vi "S2C_PCIe7841_Proc_GetClusterValues.vi"(4 "LabelText":string, 6 "Cmd In":string, 8 "Error In":errorcluster, 9 "CtrlRef":refnum<vi>) -> (0 "Error Out":errorcluster, 1 "Cmd Out":string, 2 "Send?":bool, 3 "Settings":string[][](array[string]))   [LabVIEW 2015]
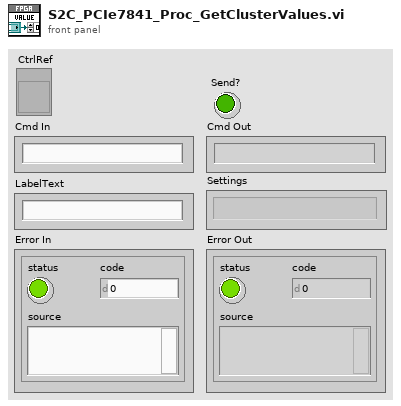
[diagram p1: front panel]
types:
  T1 = cluster{"Bit0":bool, "Bit1":bool, "Bit2":bool, "Bit3":bool, "Bit4":bool, "Bit5":bool, "Bit6":bool, "Bit7":bool, "Send":bool, "Size":bool, "State":bool}
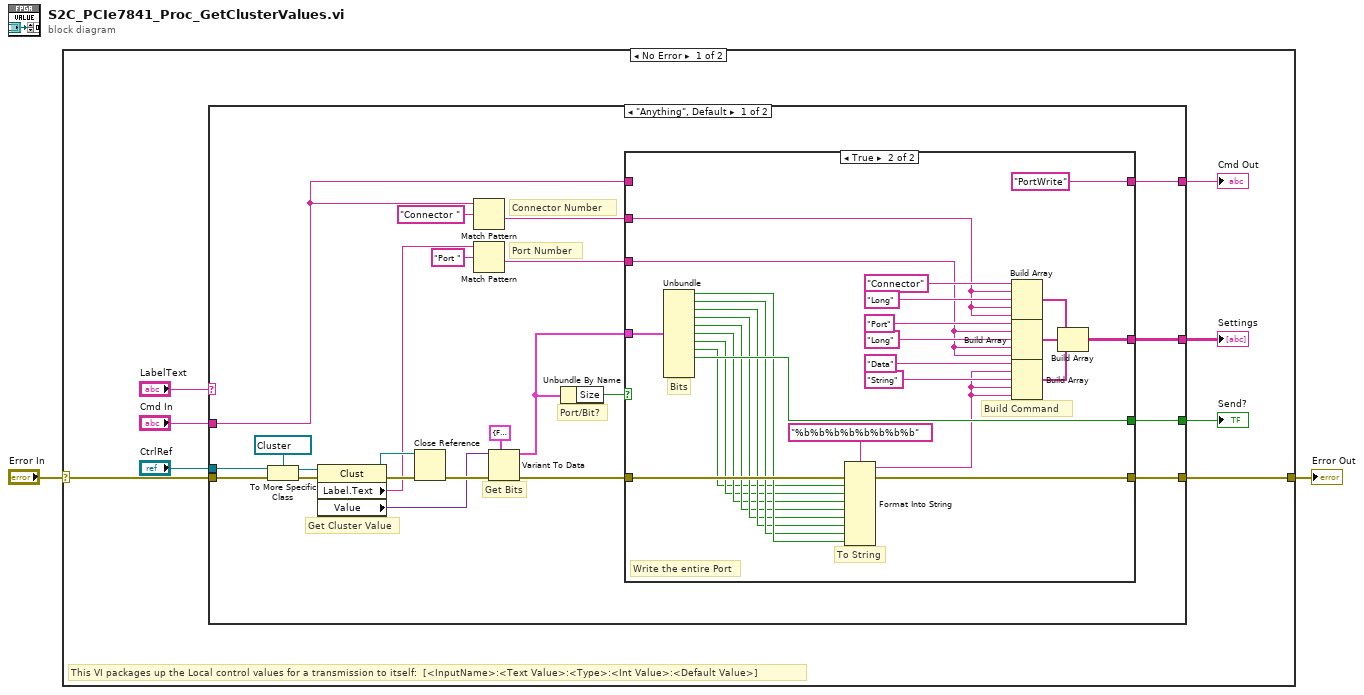
[diagram p0: block diagram]
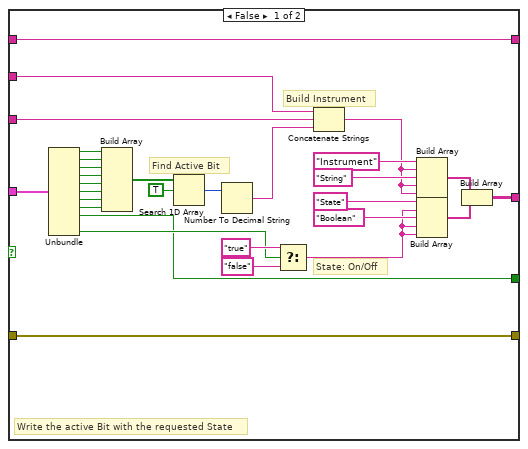
[diagram p2: hidden frame]
diagram:
  n1 = case shown="No Error" "Error In" {
    selector: "Error In" -> [w9 w92]
    tunnel: [w10 w92] -> w1
    frame No Error {
      # "This VI packages up the Local control values for a transmission to itself:  [<InputName>:<Text Value>:<Type>:<Int Value>:<Default Value>]"
      n2 = case shown="\"Anything\", Default" "LabelText" {
        tunnel: [w13 w91] -> w10
        tunnel: w9 -> [w33 w91]
        tunnel: "CtrlRef" -> [w32 _]
        tunnel: [w18 _] -> w7
        tunnel: [w17 _] -> w6
        tunnel: "Cmd In" -> [w12 _]
        tunnel: [w11 _] -> w3
        frame "Anything", Default {
          # "Port/Bit?"
          # "Get Bits"
          # "Connector Number"
          # "Port Number"
          # "Get Cluster Value"
          n3 = To More Specific Class(target class=refnum<vi> refnum ("reference"), reference=w32, error in=w33) -> (specific class reference=w30:refnum<vi>, error out=w31:errorcluster)
          n4 = property class="Clust"(reference=w30, error in=w31) -> (reference out=w28:refnum<vi>, error out=w29:errorcluster, "Label.Text"=w24:string, "Value"=w25:variant)
          n5 = Close Reference(reference=w28, error in (no error)=w29) -> (error out=w26:errorcluster)
          n6 = Match Pattern(string=w12, regular expression="Connector ") -> (after substring=w20:string)  [unwired: 1 in, 3 out]
          n7 = Match Pattern(string=w24, regular expression="Port ") -> (after substring=w19:string)  [unwired: 1 in, 3 out]
          n8 = Variant To Data(error in=w26, type=T1 {"Bit0"=FALSE, "Bit1"=FALSE, "Bit2"=FALSE, "Bit3"=FALSE, "Bit4"=FALSE, "Bit5"=FALSE, "Bit6"=FALSE, "Bit7"=FALSE, "Send"=FALSE, "Size"=FALSE, "State"=FALSE} ("Port 1"), Variant=w25) -> (data=w16:T1, error out=w14:errorcluster)
          n9 = Unbundle By Name(w16) -> ("Size"=w15:bool)
          n10 = case shown="True" w15 {
            tunnel: w16 -> [w62 w89]
            tunnel: w20 -> [w34 w82]
            tunnel: w19 -> [w35 w81]
            tunnel: [w40 w84] -> w18
            tunnel: [w38 w83] -> w17
            tunnel: w14 -> [w37 w78]
            tunnel: [w37 w76] -> w13
            tunnel: w12 -> [w36 _]
            tunnel: [w36 "PortWrite" ("Cmd In")] -> w11
            frame False {
              # "Write the active Bit with the requested State"
              # "State: On/Off"
              # "Find Active Bit"
              # "Build Instrument"
              n11 = Unbundle(w62) -> ("Bit0"=w54:bool, "Bit1"=w55:bool, "Bit2"=w56:bool, "Bit3"=w57:bool, "Bit4"=w58:bool, "Bit5"=w59:bool, "Bit6"=w60:bool, "Bit7"=w61:bool, "Send"=w38:bool, "State"=w39:bool)  [unwired: 1 out]
              n12 = Build Array(w54, w55, w56, w57, w58, w59, w60, w61) -> (w53:bool[])
              n13 = Search 1D Array(1D array=w53, element=TRUE) -> (index of element=w51:i32)  [unwired: 1 in]
              n14 = Number To Decimal String(number=w51) -> (decimal integer string=w50:string)  [unwired: 1 in]
              n15 = Select(t="true", s=w39, f="false") -> (s? t:f=w43:string)
              n16 = Concatenate Strings(w34, w35, w50) -> (w48:string)
              n17 = Build Array("Instrument" ("element"), w48, "String" ("element"), w48, w48) -> (w42:string[])
              n18 = Build Array("State" ("element"), w43, "Boolean" ("element"), w43, w43) -> (w41:string[])
              n19 = Build Array(w42, w41) -> (w40:string[][])
            }
            frame True {
              # "Write the entire Port"
              # "Build Command"
              # "To String"
              # "Bits"
              n20 = Unbundle(w89) -> ("Bit0"=w71:bool, "Bit1"=w70:bool, "Bit2"=w69:bool, "Bit3"=w68:bool, "Bit4"=w67:bool, "Bit5"=w66:bool, "Bit6"=w65:bool, "Bit7"=w64:bool, "Send"=w83:bool)  [unwired: 2 out]
              n21 = Format Into String(format string="%b%b%b%b%b%b%b%b", error in=w78, w64, w65, w66, w67, w68, w69, w70, w71) -> (resulting string=w75:string, error out=w76:errorcluster)  [unwired: 1 in]
              n22 = Build Array("Connector" ("element"), w82, "Long" ("element"), w82, w82) -> (w85:string[])
              n23 = Build Array("Port" ("element"), w81, "Long" ("element"), w81, w81) -> (w73:string[])
              n24 = Build Array("Data" ("element"), w75, "String" ("element"), w75, w75) -> (w72:string[])
              n25 = Build Array(w85, w73, w72) -> (w84:string[][])
            }
          }
        }
        frame "P1C1Exe".."P8C8Exe" {
          # "This case handles the \"Execute\" buttons"
        }
      }
      "Settings" <- w7
      "Send?" <- w6
      "Cmd Out" <- w3
    }
    frame Error {
    }
  }
  "Error Out" <- w1
